vi "Read wavelength1.vi"(8 "error in (no error)":errorcluster, 11 "ADCWavelength in":refnum<class "ADCWavelength.lvclass">) -> (0 "error out":errorcluster, 2 "wavelength1":dbl[unit]=3e-07 min=3e-07 max=9.999999999999999e-06, 3 "ADCWavelength out":refnum<class "ADCWavelength.lvclass">)   [LabVIEW 2014, in "TCSDataDefinitions.lvlib" / "TCSAtmosphericDispersionCommand.lvlib" / "ADCWavelength.lvclass"]
uses:
  ADCWavelength.lvclass
  ADCWavelength.lvclass/ADCWavelength.ctl
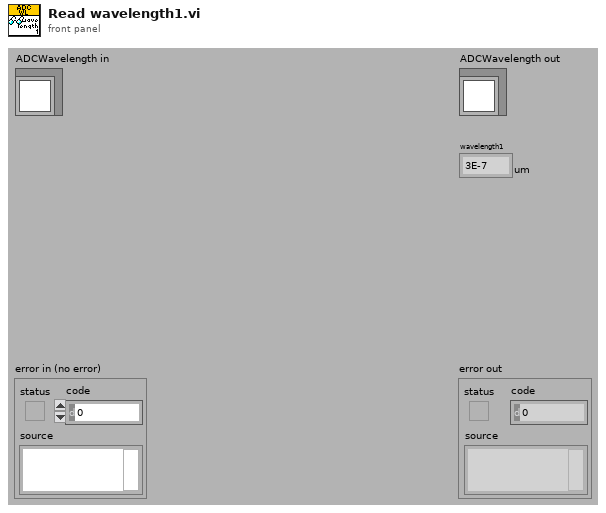
[diagram p1: front panel]
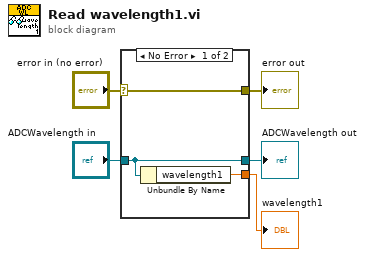
[diagram p0: block diagram]
diagram:
  n1 = case shown="No Error" "error in (no error)" {
    selector: "error in (no error)" -> [w8 w9]
    tunnel: [w8 w9] -> w4
    tunnel: [w7 w10] -> w2
    tunnel: "ADCWavelength in" -> [w7 w10]
    tunnel: [w6 _] -> w1
    frame No Error {
      n2 = Unbundle By Name(w7) -> ("wavelength1"=w6:dbl[unit])
    }
    frame Error {
    }
  }
  "error out" <- w4
  "ADCWavelength out" <- w2
  "wavelength1" <- w1
